vi "XIPIN_AXI_Bridge_for_PCI_Express_Gen3_Subsystem_2_0.vi"   [LabVIEW 2017]
doc: "The Advanced eXtensible Interface (AXI) Bridge for Gen3 PCI Express is an interface between the AXI4 and PCI Express\n------------------------------------\n<b>Need License</b> : No\n<b>Interface</b> : AXI4"
uses:
  <vilib>/rvi/XilinxIP/XIPIN_XNode/niFpgaXIPIN.xnode
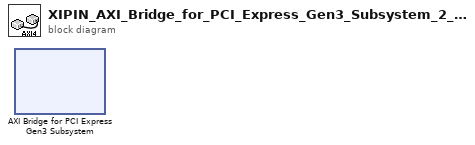
[diagram p0: block diagram]
diagram:
  n1 = xnode ("AXI Bridge for PCI Express Gen3 Subsystem")() -> ()
